vi "NPL Joerger ADC Convert.vi"(11 "Input":ext[][](array[numeric])) -> (3 "Output":ext[][](array[numeric]))   [LabVIEW 2013]
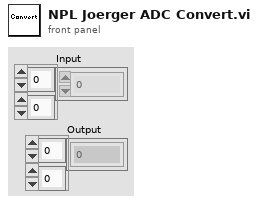
[diagram p1: front panel]
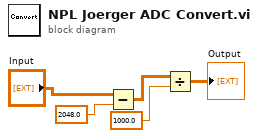
[diagram p0: block diagram]
diagram:
  n1 = Subtract(x="Input", y=2048.0) -> (x-y=w3:ext[][])
  n2 = Divide(x=w3, y=1000.0) -> (x/y=→"Output":ext[][])
